vi "comm set default config.vi"(8 "error in (no error)":errorcluster, 10 "options string":string, 11 "serial port name":string) -> (0 "error out":errorcluster)   [LabVIEW 2017, in "lvserial.lvlib"]
doc: "Ssets the default configuration for a communications device"
uses:
  lvserial.lvlib
  lvserial.dll
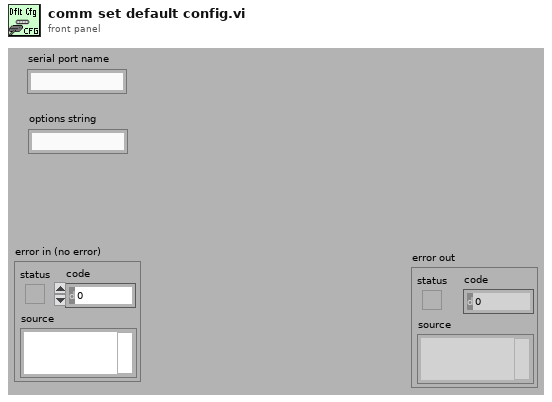
[diagram p1: front panel]
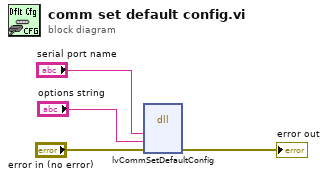
[diagram p0: block diagram]
diagram:
  n1 = dll-call lib="lvserial.dll" fn="lvCommSetDefaultConfig"("shPort"="serial port name", "shOptions"="options string", "error in (no error)"="error in (no error)") -> ("error in (no error)"=→"error out":errorcluster)  [unwired: 5 in, 3 out]
